vi "connect to server.vi"(8 "Delay Time (s)":dbl=4.0, 10 "name or relative path":string="TestScripts", 11 "Sequence path":path=path "C:/Func Jobs/SnapOn/ModisEdge/Scanner/Test Sequence/ModisEdgeScanner.seq") -> (3 "Pass":bool)   [LabVIEW 2015]
panel:
  out "standard output 2":string
  out "error out":errorcluster
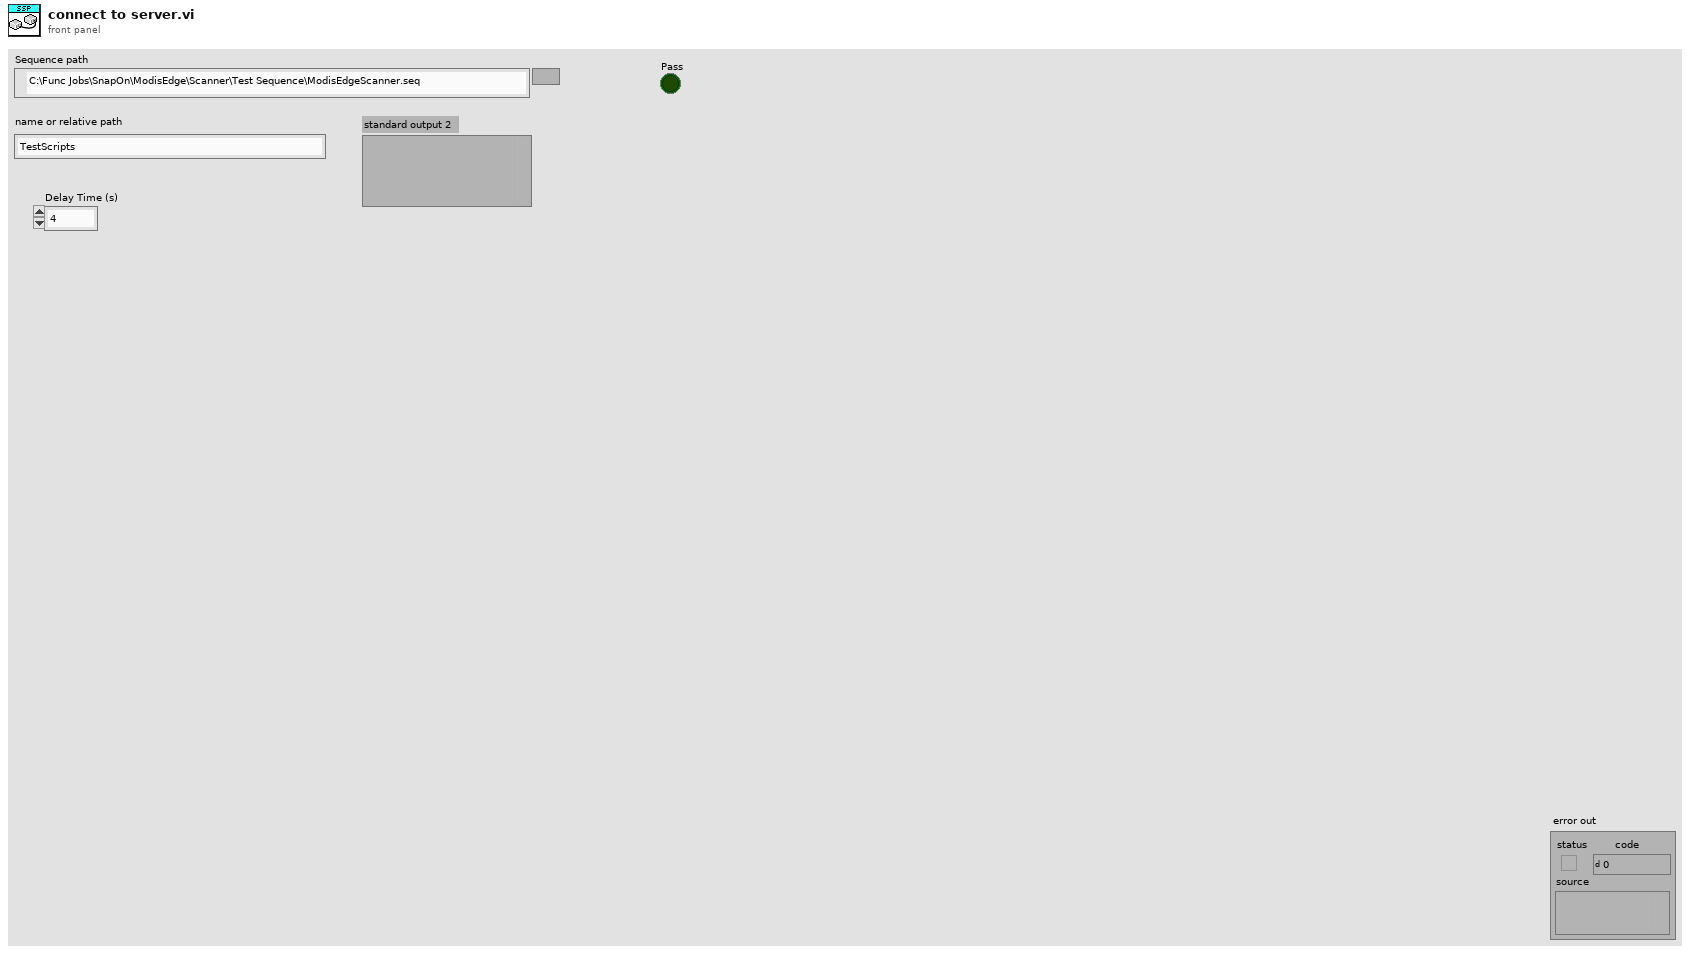
[diagram p1: front panel]
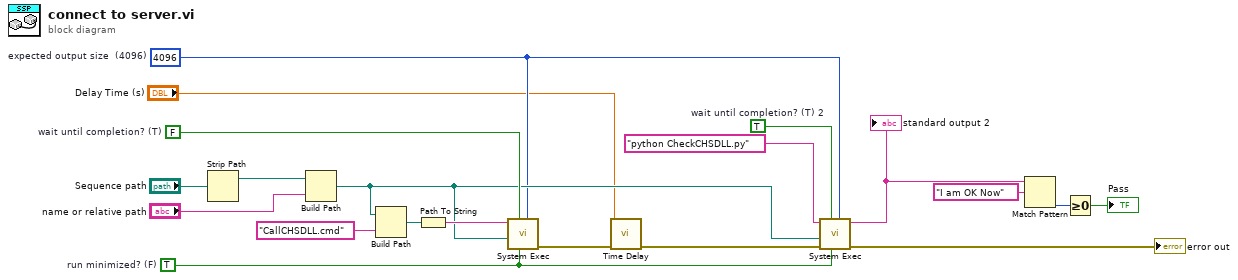
[diagram p0: block diagram]
diagram:
  w7 = TRUE  # run minimized? (F)
  w10 = TRUE  # wait until completion? (T) 2
  w20 = FALSE  # wait until completion? (T)
  w9 = u32 4096  # expected output size  (4096)
  n1 = Strip Path(path="Sequence path") -> (stripped path=w14:path)  [unwired: 1 out]
  n2 = Build Path(base path=w14, name or relative path="name or relative path") -> (appended path=w11:path)
  n3 = Build Path(base path=w11, name or relative path="CallCHSDLL.cmd" ("Command")) -> (appended path=w17:path)
  n4 = Path To String(path=w17) -> (string=w16:string)
  n5 = call <vilib>:"System Exec.vi"("expected output size  (4096)"=w9, "run minimized? (F)"=w7, "wait until completion? (T)"=w20, "working directory"=w11, "command line"=w16) -> ("error out"=w13:errorcluster)  [unwired: 3 in, 3 out]
  n6 = call "Time Delay"("error in (no error)"=w13, "Delay Time (s)"="Delay Time (s)") -> ("error out"=w2:errorcluster)  [unwired: 9 in]
  n7 = call <vilib>:"System Exec.vi"("expected output size  (4096)"=w9, "run minimized? (F)"=w7, "wait until completion? (T)"=w10, "error in (no error)"=w2, "working directory"=w11, "command line"="python CheckCHSDLL.py") -> ("error out"=→"error out":errorcluster, "standard output"=w6:string)  [unwired: 2 in, 2 out]
  "standard output 2" <- w6
  n8 = Match Pattern(string=w6, regular expression="I am OK Now") -> (offset past match=w4:i32)  [unwired: 1 in, 3 out]
  n9 = Greater Or Equal To 0?(x=w4) -> (x >= 0?=→"Pass":bool)
